vi "Configure Heater Output.vi"(0 "VISA resource name":refnum<visa-resource-name>, 1 "Mode (0:Off)":u16(ring) items=["Off", "Closed Loop PID", "Zone", "Open Loop"], 2 "Power Up Enable (F: Off)":bool, 5 "Heater Output (1:1)":u16(ring)=1 items=["1"=1, "2"=2], 7 "Input (0:None)":u16(ring) items=["None", "A", "B", "C", "D"], 9 "Max Current (0:User Specified)":u16(ring) items=["User Specified", "0.707 A", "1.0 A", "1.141 A", "2.0 A"], 11 "error in (no error)":errorcluster, 12 "Heater Out Display (1:Current)":u16(ring)=1 items=["Current"=1, "Power"=2], 13 "Max User Current (2.000)":dbl=2.0 format="%.3f", 14 "Heater Resistance (1:25 Ohms)":u16(ring)=1 items=["25 Ohms"=1, "50 Ohms"=2]) -> (4 "VISA resource name out":refnum<visa-resource-name>, 15 "error out":errorcluster)   [LabVIEW 2024, in "Lake Shore 336.lvlib"]
doc: "This VI configures the heater outputs. Heater outputs, 1 and 2, are traditional control loop heater outputs for a cryogenic temperature controller. The two outputs are identical except in the amount of power available. Output 1 can provide up to 100 W, and output 2 can provide up to 50 W."
uses:
  Lake Shore 336.lvlib
  Instance           1 31Saved   Configure Heater Output .vi
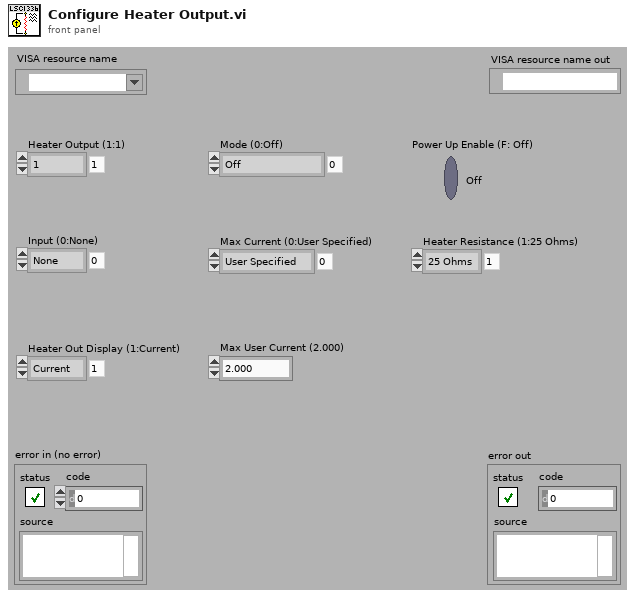
[diagram p1: front panel]
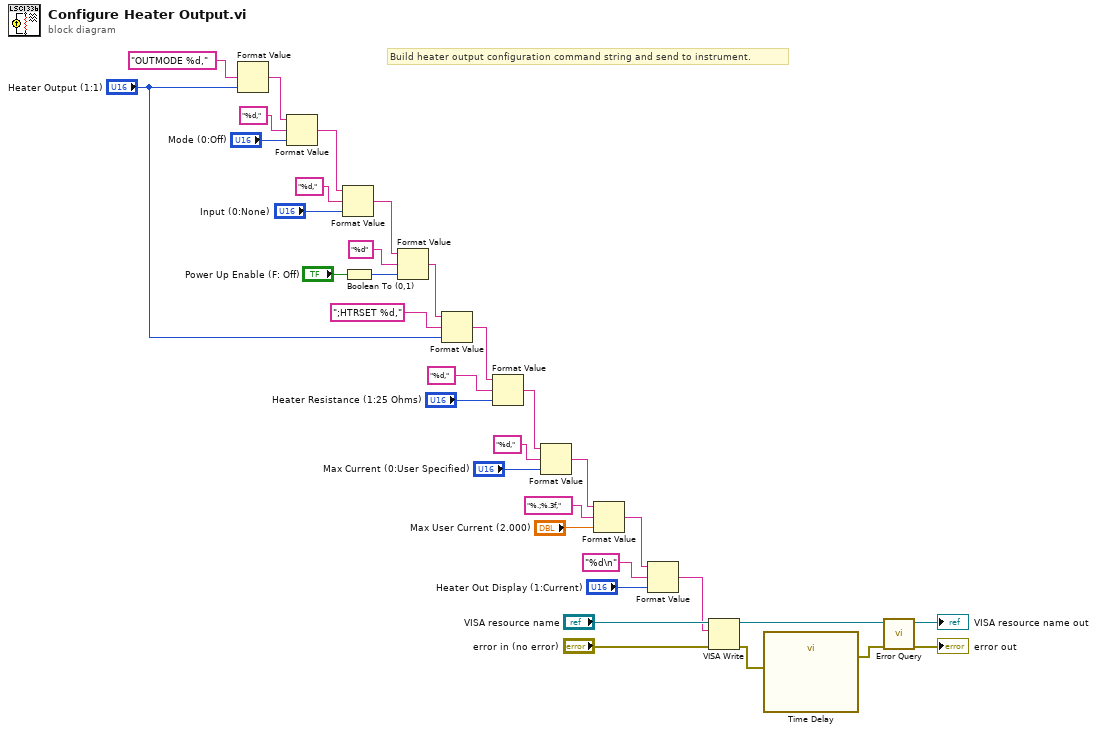
[diagram p0: block diagram]
diagram:
  # "Build heater output configuration command string and send to instrument."
  n1 = Format Value(format string="OUTMODE %d,", value (0)="Heater Output (1:1)") -> (output string=w4:string)  [unwired: 1 in]
  n2 = Format Value(string ("")=w4, format string="%d,", value (0)="Mode (0:Off)") -> (output string=w11:string)
  n3 = Format Value(string ("")=w11, format string="%d,", value (0)="Input (0:None)") -> (output string=w10:string)
  n4 = Boolean To (0,1)(Boolean="Power Up Enable (F: Off)") -> (0, 1=w24:i16)
  n5 = Format Value(string ("")=w10, format string="%d", value (0)=w24) -> (output string=w3:string)
  n6 = Format Value(string ("")=w3, format string=";HTRSET %d,", value (0)="Heater Output (1:1)") -> (output string=w2:string)
  n7 = Format Value(string ("")=w2, format string="%d,", value (0)="Heater Resistance (1:25 Ohms)") -> (output string=w9:string)
  n8 = Format Value(string ("")=w9, format string="%d,", value (0)="Max Current (0:User Specified)") -> (output string=w16:string)
  n9 = Format Value(string ("")=w16, format string="%.;%.3f,", value (0)="Max User Current (2.000)") -> (output string=w8:string)
  n10 = Format Value(string ("")=w8, format string="%d\n", value (0)="Heater Out Display (1:Current)") -> (output string=w7:string)
  n11 = VISA Write(VISA resource name="VISA resource name", write buffer=w7, error in (no error)="error in (no error)") -> (VISA resource name out=w32:refnum<visa-resource-name>, error out=w28:errorcluster)  [unwired: 1 out]
  n12 = call "Time Delay"("error in (no error)"=w28) -> ("error out"=w27:errorcluster)  [unwired: 10 in]
  n13 = call "Error Query.vi"("error in (no error)"=w27, "VISA resource name"=w32) -> ("error out"=→"error out":errorcluster, "VISA resource name out"=→"VISA resource name out":refnum<visa-resource-name>)  [unwired: 7 in, 1 out]
